vi "test Bad Regex.vi"(8 "error in":errorcluster) -> (0 "error out":errorcluster)   [LabVIEW 2024, in "serenial.io-ase.test.lvlib"]
uses:
  serenial.io-ase.test.lvlib
  <vilib>/addons/_JKI Toolkits/Caraya/classes/Test/Test.lvclass
  <vilib>/addons/_JKI Toolkits/Caraya/classes/Assert/Assert.lvclass
  serenial.io-ase/ase/ase.lvclass
  <vilib>/addons/_JKI Toolkits/Caraya/classes/Assert/Assert Equal Value and Type_Variant.vi
  serenial.io-ase/ase/Start Call (Exe-Args).vi
  Bad Regex/Bad Regex.lvclass
  Bad Regex/Bad Value.ctl
  C:/Users/marc/code/sift-streaming/labview/Sift/Dependencies/asynchronous-system-exec-v2.0.0/serenial.io-ase/configuration/configuration.lvclass
  C:/Users/marc/code/sift-streaming/labview/Sift/Dependencies/asynchronous-system-exec-v2.0.0/serenial.io-ase.test/Bad Regex/Bad Regex.lvclass
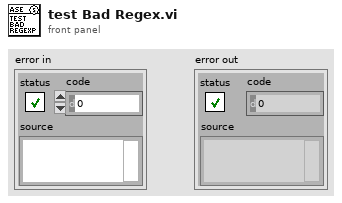
[diagram p1: front panel]
types:
  T1 = typedef "serenial.io-ase.test.lvlib/Bad Regex.lvclass/Bad Value.ctl" = enum16{"Out", "Err", "Both"}
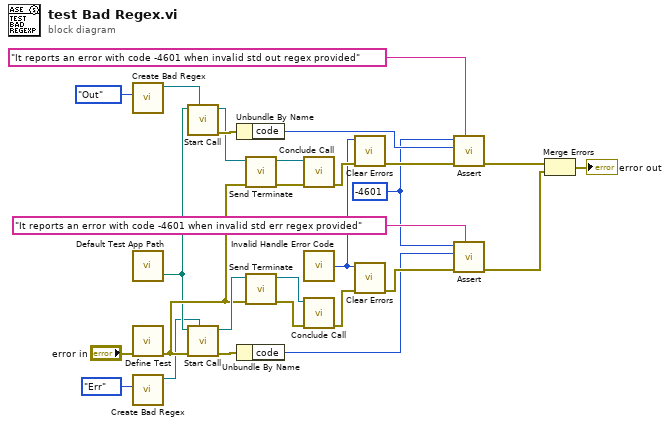
[diagram p0: block diagram]
diagram:
  w7 = -4601 ("code")
  n1 = call "Create Bad Regex.vi"("Bad Value"=Bad_Value."Out") -> ("Bad Regex out"=w4:refnum<class "Bad Regex.lvclass">)  [unwired: 9 in, 1 out]
  n2 = call "Default Test App Path.vi"() -> ("Exe Path"=w5:path)  [unwired: 2 in, 1 out]
  n3 = call <vilib>:"Define Test.vi"("error in (no error)"="error in") -> ("error out"=w8:errorcluster)  [unwired: 9 in, 1 out]
  n4 = call "Create Bad Regex.vi"("Bad Value"=Bad_Value."Err") -> ("Bad Regex out"=w1:refnum<class "Bad Regex.lvclass">)  [unwired: 9 in, 1 out]
  n5 = call-poly "Start Call.vi"("Configuration"=w4, "Executable Path"=w5) -> ("error out"=w20:errorcluster, "New ASE Handle"=w19:refnum<class "ase.lvclass">)  [unwired: 8 in]
  n6 = call-poly "Start Call.vi"("Configuration"=w1, "error in"=w8, "Executable Path"=w5) -> ("error out"=w17:errorcluster, "New ASE Handle"=w18:refnum<class "ase.lvclass">)  [unwired: 7 in]
  n7 = Unbundle By Name(w20) -> ("code"=w26:i32)
  n8 = Unbundle By Name(w17) -> ("code"=w12:i32)
  n9 = call "Send Terminate.vi"("error in"=w8, "ASE Handle"=w19) -> ("error out"=w21:errorcluster, "ASE Handle Duplicate"=w22:refnum<class "ase.lvclass">)  [unwired: 7 in, 1 out]
  n10 = call "Send Terminate.vi"("error in"=w8, "ASE Handle"=w18) -> ("error out"=w16:errorcluster, "ASE Handle Duplicate"=w15:refnum<class "ase.lvclass">)  [unwired: 7 in, 1 out]
  n11 = call "Conclude Call.vi"("error in"=w21, "ASE Handle"=w22) -> ("error out"=w25:errorcluster)  [unwired: 7 in, 2 out]
  n12 = call "Invalid Handle Error Code.vi"() -> ("Invalid Handle Error"=w6:i32)
  n13 = call "Conclude Call.vi"("error in"=w16, "ASE Handle"=w15) -> ("error out"=w13:errorcluster)  [unwired: 7 in, 2 out]
  n14 = call <vilib>:"Clear Errors.vi"("error in (no error)"=w25, "specific error code to clear (0: all)"=w6) -> ("error out"=w23:errorcluster)  [unwired: 4 in, 1 out]
  n15 = call <vilib>:"Clear Errors.vi"("error in (no error)"=w13, "specific error code to clear (0: all)"=w6) -> ("error out"=w14:errorcluster)  [unwired: 4 in, 1 out]
  n16 = call-poly <vilib>:"Assert.vi"("Label"="It reports an error with code -4601 when invalid std out regex provided", "error in (no error)"=w23, "Y"=w26, "X"=w7) -> ("error out"=w24:errorcluster)  [unwired: 6 in, 1 out]
  n17 = call-poly <vilib>:"Assert.vi"("Label"="It reports an error with code -4601 when invalid std err regex provided", "error in (no error)"=w14, "Y"=w12, "X"=w7) -> ("error out"=w10:errorcluster)  [unwired: 6 in, 1 out]
  n18 = Merge Errors(w24, w10) -> (→"error out":errorcluster)
